vi "Shutdown.vi"(11 "Connection Handler in":refnum<class "Connection Handler.lvclass">) -> ()   [LabVIEW 2017, in "Network Interface.lvlib" / "Connection Handler.lvclass"]
uses:
  <vilib>/gpm_packages/@cs/Network-sink/Source/Network Interface/Connection Handler/Connection Handler.lvclass
  <vilib>/gpm_packages/@cs/Network-sink/Source/Network Interface/Connection Handler/Connection Handler.lvclass/Connection Handler.ctl
  <vilib>/gpm_packages/@cs/Network-sink/Source/Network Interface/Connection Handler/Synchronous Write Request.ctl
  <vilib>/gpm_packages/@cs/Network-sink/Source/Network Interface/Message Queue/Message Queue.lvclass/Message Queue.ctl
  b29d0aad-a3f0-49c2-a7fb-3f3b968fec31.vi
  <vilib>/gpm_packages/@cs/Network-sink/Source/Network Interface/Message Queue/Protected Enqueue.vi
  <vilib>/Utility/error.llb/Error Cluster From Error Code.vi
  <vilib>/gpm_packages/@cs/Network-sink/Source/Network Interface/IConnection/IConnection.lvclass
  <vilib>/ErrorRing/Error Ring.xnode
  <vilib>/gpm_packages/@cs/Network-sink/Source/Network Interface/Message Queue/Message Queue.lvclass
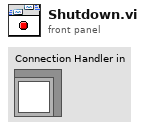
[diagram p1: front panel]
types:
  T1 = typedef "Network Interface.lvlib/Message Queue.lvclass/Message Cluster.ctl" = cluster{"Msg":string, "Data":variant}
  T2 = typedef "Network Interface.lvlib/Connection Handler.lvclass/Synchronous Write Request.ctl" = cluster{"Data To Write":string, "Return Queue":refnum<queue>}
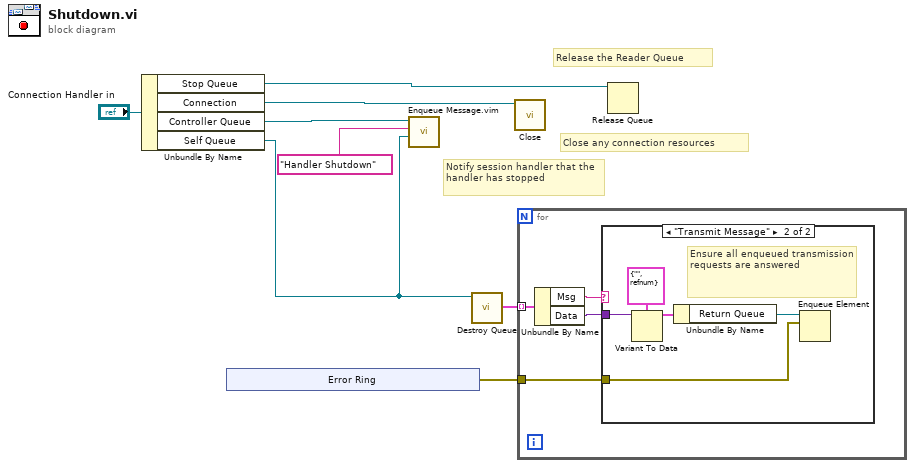
[diagram p0: block diagram]
diagram:
  # "Release the Reader Queue"
  # "Close any connection resources"
  # "Notify session handler that the handler has stopped"
  n1 = Unbundle By Name("Connection Handler in") -> ("Stop Queue"=w1:refnum<queue>, "Connection"=w3:refnum<class "IConnection.lvclass">, "Controller Queue"=w5:refnum<class "Message Queue.lvclass">, "Self Queue"=w4:refnum<class "Message Queue.lvclass">)
  n2 = xnode "Error Ring"() -> ("error out"=w2:errorcluster)
  n3 = call "Enqueue Message.vim"("Data"=w4, "Msg"="Handler Shutdown", "Message Queue in"=w5) -> ()  [unwired: 7 in, 2 out]
  n4 = call <vilib>:"Destroy Queue.vi"("Message Queue in"=w4) -> ("Remaining Elements"=w7:T1[])  [unwired: 8 in, 2 out]
  n5 = call-dynamic "Close.vi"("IConnection in"=w3) -> ()  [unwired: 10 in, 1 out]
  n6 = for {
    tunnel: w7 -> [w12] mode=indexing
    tunnel: w2 -> [w9]
    n7 = Unbundle By Name(w12) -> ("Msg"=w11:string, "Data"=w10:variant)
    n8 = case shown="\"Transmit Message\"" w11 {
      tunnel: w10 -> [_ w16]
      tunnel: w9 -> [_ w13]
      frame Default {
        # "Ignore other messages"
      }
      frame "Transmit Message" {
        # "Ensure all enqueued transmission requests are answered"
        n9 = Variant To Data(type=T2 {"Data To Write"="", "Return Queue"=refnum} ("Write Request"), Variant=w16) -> (data=w15:T2)  [unwired: 1 in, 1 out]
        n10 = Unbundle By Name(w15) -> ("Return Queue"=w14:refnum<queue>)
        n11 = Enqueue Element(queue=w14, element=w13) -> ()  [unwired: 2 in, 3 out]
      }
    }
  }
  n12 = Release Queue(queue=w1) -> ()  [unwired: 2 in, 3 out]
